vi "Handle Message.vi"(5 "Stack ID":u8, 7 "Function ID":u8, 8 "error in (no error)":errorcluster, 10 "Data":string, 11 "Distance IR Bricklet in":refnum<class "Distance IR Bricklet.lvclass">) -> (0 "error out":errorcluster, 1 "Send Answer":bool, 2 "Answer":variant, 3 "Distance IR Bricklet out":refnum<class "Distance IR Bricklet.lvclass">)   [LabVIEW 2011, in "Tinkerforge.lvlib" / "Distance IR Bricklet.lvclass"]
doc: "This VI is the child implementation of \"Handle Message.vi\" and processes all responses for this device type."
uses:
  Distance IR Bricklet.lvclass
  Distance IR Bricklet.lvclass/Distance IR Bricklet.ctl
  Device/Device.lvclass
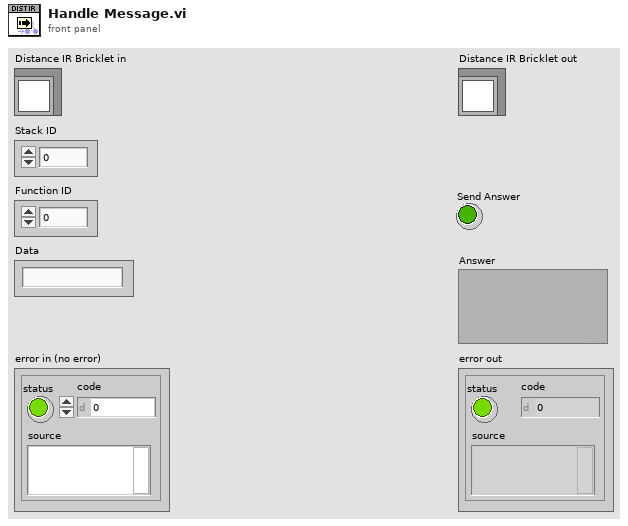
[diagram p1: front panel]
types:
  T1 = typedef "Tinkerforge.lvlib/Device.lvclass/Callback Threshold.ctl" = cluster{"Callback Option":T2, "min":i16, "max":i16}
  T2 = typedef "Tinkerforge.lvlib/Device.lvclass/Callback Option.ctl" = enum8{"CB off", "outside range", "inside range", "smaller", "greater"}
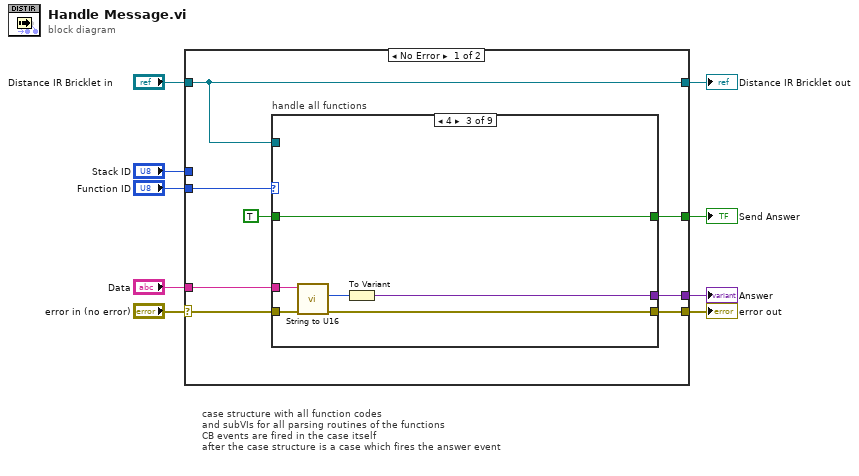
[diagram p0: block diagram]
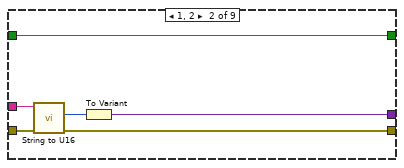
[diagram p3: hidden frame]
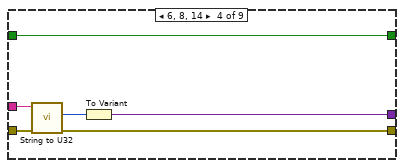
[diagram p4: hidden frame]
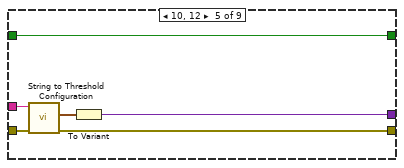
[diagram p5: hidden frame]
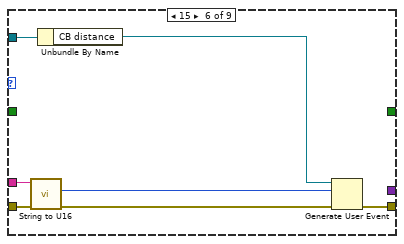
[diagram p6: hidden frame]
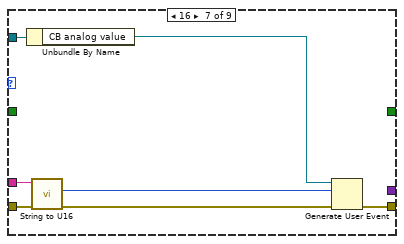
[diagram p7: hidden frame]
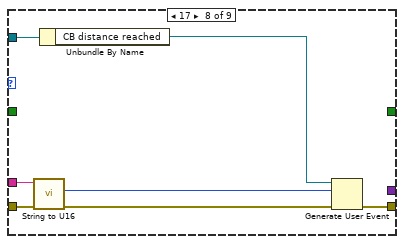
[diagram p8: hidden frame]
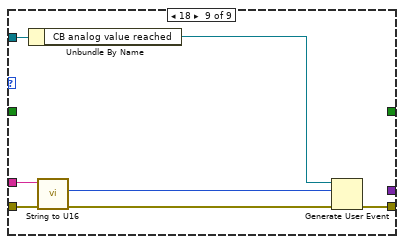
[diagram p9: hidden frame]
diagram:
  # "case structure with all function codes\nand subVIs for all parsing routines of the functions\nCB events are fired in the case itself\nafter the case structure is a case which fires the answer event"
  n1 = case shown="No Error" "error in (no error)" {
    selector: "error in (no error)" -> [w13 w70]
    tunnel: "Distance IR Bricklet in" -> [w17 w71]
    tunnel: "Stack ID" -> [_ _]
    tunnel: "Function ID" -> [w16 _]
    tunnel: "Data" -> [w14 _]
    tunnel: [w17 w71] -> w4
    tunnel: [w11 w70] -> w3
    tunnel: [w12 _] -> w2
    tunnel: [w10 _] -> w1
    frame No Error {
      n2 = case "handle all functions" shown="4" w16 {
        tunnel: w13 -> [_ w21 w27 w33 w39 w45 w52 w59 w66]
        tunnel: w14 -> [_ w20 w24 w32 w37 w44 w51 w58 w65]
        tunnel: TRUE -> [_ w23 w29 w35 w41 _ _ _ _]
        tunnel: [_ w23 w29 w35 w41 _ _ _ _] -> w10
        tunnel: [_ w19 w26 w31 w38 w46 w53 w60 w67] -> w11
        tunnel: [_ w22 w28 w34 w40 _ _ _ _] -> w12
        tunnel: w17 -> [_ _ _ _ _ w48 w55 w62 w69]
        frame Default {
          # "nothing to do"
        }
        frame 1, 2 {
          n3 = call "String to U16.vi"("Error In"=w21, "String"=w20) -> ("Error Out"=w19:errorcluster, "U16"=w18:u16)  [unwired: 7 in, 1 out]
          n4 = To Variant(anything=w18) -> (Variant=w22:variant)
        }
        frame 4 {
          n5 = call "String to U16.vi"("Error In"=w27, "String"=w24) -> ("Error Out"=w26:errorcluster, "U16"=w25:u16)  [unwired: 7 in, 1 out]
          n6 = To Variant(anything=w25) -> (Variant=w28:variant)
        }
        frame 6, 8, 14 {
          n7 = call "String to U32.vi"("Error In"=w33, "String"=w32) -> ("Error Out"=w31:errorcluster, "U32"=w30:u32)  [unwired: 7 in, 1 out]
          n8 = To Variant(anything=w30) -> (Variant=w34:variant)
        }
        frame 10, 12 {
          n9 = call "String to Threshold Configuration.vi"("Error In"=w39, "String"=w37) -> ("Error Out"=w38:errorcluster, "Callback Threshold"=w36:T1)  [unwired: 7 in, 1 out]
          n10 = To Variant(anything=w36) -> (Variant=w40:variant)
        }
        frame 15 {
          n11 = call "String to U16.vi"("Error In"=w45, "String"=w44) -> ("Error Out"=w43:errorcluster, "U16"=w42:u16)  [unwired: 7 in, 1 out]
          n12 = Unbundle By Name(w48) -> ("CB distance"=w47:refnum<user-event>)
          n13 = Generate User Event(user event=w47, event data cluster=w42, error in=w43) -> (error out=w46:errorcluster)  [unwired: 1 out]
        }
        frame 16 {
          n14 = Unbundle By Name(w55) -> ("CB analog value"=w54:refnum<user-event>)
          n15 = call "String to U16.vi"("Error In"=w52, "String"=w51) -> ("Error Out"=w49:errorcluster, "U16"=w50:u16)  [unwired: 7 in, 1 out]
          n16 = Generate User Event(user event=w54, event data cluster=w50, error in=w49) -> (error out=w53:errorcluster)  [unwired: 1 out]
        }
        frame 17 {
          n17 = call "String to U16.vi"("Error In"=w59, "String"=w58) -> ("Error Out"=w56:errorcluster, "U16"=w57:u16)  [unwired: 7 in, 1 out]
          n18 = Unbundle By Name(w62) -> ("CB distance reached"=w61:refnum<user-event>)
          n19 = Generate User Event(user event=w61, event data cluster=w57, error in=w56) -> (error out=w60:errorcluster)  [unwired: 1 out]
        }
        frame 18 {
          n20 = Unbundle By Name(w69) -> ("CB analog value reached"=w68:refnum<user-event>)
          n21 = call "String to U16.vi"("Error In"=w66, "String"=w65) -> ("Error Out"=w64:errorcluster, "U16"=w63:u16)  [unwired: 7 in, 1 out]
          n22 = Generate User Event(user event=w68, event data cluster=w63, error in=w64) -> (error out=w67:errorcluster)  [unwired: 1 out]
        }
      }
    }
    frame Error {
    }
  }
  "error out" <- w3
  "Distance IR Bricklet out" <- w4
  "Answer" <- w2
  "Send Answer" <- w1
